vi "MSGR Handshake.vi"(0 "MSGR Q name":T2, 5 "Msg":string, 9 "Parameters":string, 11 "error in (no error)":errorcluster, 12 "timeout in ms (-1)":i32=-1) -> (6 "MSGR":T1, 8 "timed out?":bool, 15 "error out":errorcluster)   [LabVIEW 2018]
doc: "$Author::Richard Jennings $\n$Rev:: $\n$Date:: May, 2008 $\n\nOVERVIEW:\nReentrant VI to receive messages via a MSGR Q. If the Q does not exist this VI will create it, then wait for data.\n\nINPUTS (Controls):\n<name> - <short description of each control wired to connector pane>\n\nOUTPUTS (Indicators):\n<name> - <short description of each indicator wired to connector pane>\n\nCopyright 2008 - 2017 Jennings Embedded Servies. All rights reserved.\nAuthor makes no warranties or guarantees related to performance of the software.\nUSE AT YOUR OWN RISK\nwww.jembedded.com\n\n\n\nMIT License\n\nCopyright (c) 2020 RichardLGP5\n\nPermission is hereby granted, free of charge, to any person obtaining a copy\nof this software and associated documentation files (the \"Software\"), to deal\nin the Software without restriction, including without limitation the rights\nto use, copy, modify, merge, publish, distribute, sublicense, and/or sell\ncopies of the Software, and to permit persons to whom the Software is\nfurnished to do so, subject to the following conditions:\n\nThe above copyright notice and this permission notice shall be included in all\ncopies or substantial portions of the Software.\n\nTHE SOFTWARE IS PROVIDED \"AS IS\", WITHOUT WARRANTY OF ANY KIND, EXPRESS OR\nIMPLIED, INCLUDING BUT NOT LIMITED TO THE WARRANTIES OF MERCHANTABILITY,\nFITNESS FOR A PARTICULAR PURPOSE AND NONINFRINGEMENT. IN NO EVENT SHALL THE\nAUTHORS OR COPYRIGHT HOLDERS BE LIABLE FOR ANY CLAIM, DAMAGES OR OTHER\nLIABILITY, WHETHER IN AN ACTION OF CONTRACT, TORT OR OTHERWISE, ARISING FROM,\nOUT OF OR IN CONNECTION WITH THE SOFTWARE OR THE USE OR OTHER DEALINGS IN THE\nSOFTWARE."
uses:
  MSGR Q Name TypeDef.ctl
  MSGR Q Data TypeDef.ctl
  MSGR Get Q.vi
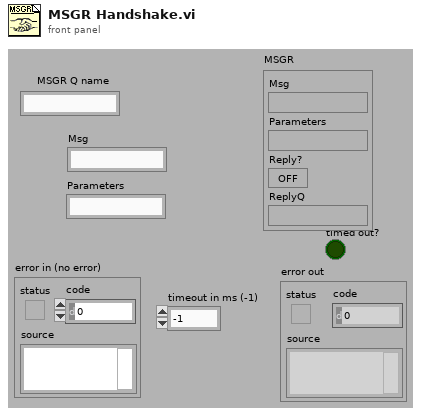
[diagram p1: front panel]
types:
  T1 = typedef "MSGR Q Data TypeDef.ctl" = cluster{"Msg":string, "Parameters":string, "Reply?":bool, "ReplyQ":string}
  T2 = typedef "MSGR Q Name TypeDef.ctl" = string
  T3 = typedef "MSGR Q Ref TypeDef.ctl" = refnum<queue>
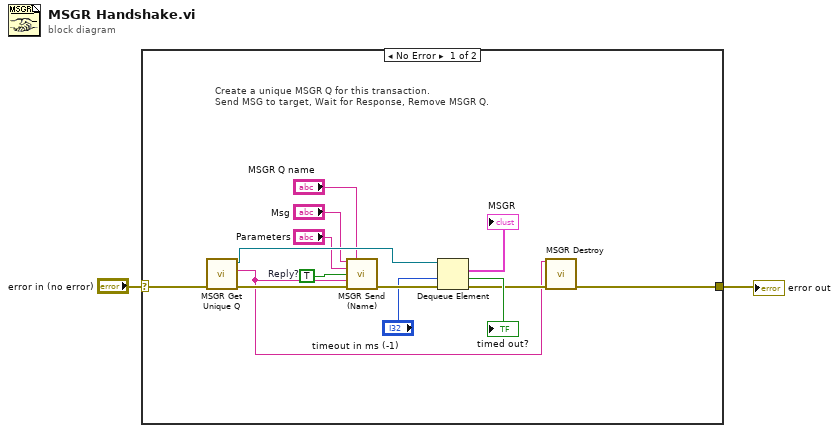
[diagram p0: block diagram]
diagram:
  n1 = case shown="No Error" "error in (no error)" {
    selector: "error in (no error)" -> [w16 w17]
    tunnel: [w7 w17] -> w2
    frame No Error {
      w15 = TRUE  # Reply?
      # "Create a unique MSGR Q for this transaction.\nSend MSG to target, Wait for Response, Remove MSGR Q."
      n2 = call "MSGR Get Unique Q.vi"("error in (no error)"=w16) -> ("error out"=w14:errorcluster, "MSGR Q name"=w6:T2, "MSG Q"=w12:T3)  [unwired: 8 in]
      n3 = call "MSGR Send (Name).vi"("Msg"="Msg", "MSGR Q name"="MSGR Q name", "Parameters"="Parameters", "Reply?"=w15, "ReplyQ"=w6, "error in (no error)"=w14) -> ("error out"=w13:errorcluster)  [unwired: 8 in, 1 out]
      n4 = Dequeue Element(queue=w12, timeout in ms (-1)="timeout in ms (-1)", error in (no error)=w13) -> (element=→"MSGR":T1, timed out?=→"timed out?":bool, error out=w8:errorcluster)  [unwired: 1 out]
      n5 = call "MSGR Destroy.vi"("MSGR Q name"=w6, "error in (no error)"=w8) -> ("error out"=w7:errorcluster)  [unwired: 13 in]
    }
    frame Error {
    }
  }
  "error out" <- w2
